vi "PadArrayPost.vi"(8 "Pad Length":i32, 11 "Input Array":dbl[](array[numeric])) -> (3 "Padded Array":dbl[](array[numeric]))   [LabVIEW 2016]
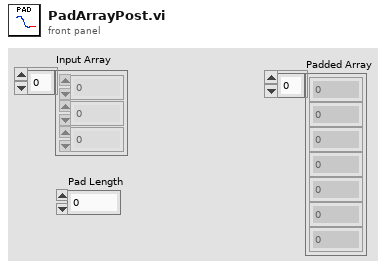
[diagram p1: front panel]
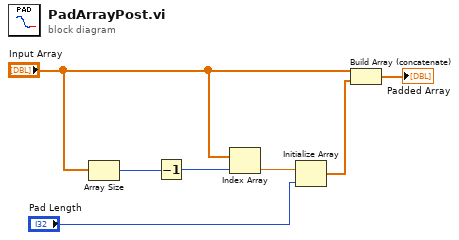
[diagram p0: block diagram]
diagram:
  n1 = Array Size(array="Input Array") -> (size(s)=w6:i32)
  n2 = Decrement(x=w6) -> (x-1=w5:i32)
  n3 = Index Array(array="Input Array", index=w5) -> (element=w4:dbl)
  n4 = Initialize Array(w4, "Pad Length") -> (w1:dbl[])
  n5 = Build Array (concatenate)("Input Array", w1) -> (→"Padded Array":dbl[])
